vi "scanDeviceStepLogic.vi"(4 "actScan":i32, 6 "actStep":i32) -> (2 "timedOut":bool)   [LabVIEW 2014]
uses:
  Controls/infoHandle.ctl
  Sequencer/trackGlobVar.vi
  scanDeviceGlobalVars.vi
  <vilib>/rvi/Emulation/niFpgaGetClockAttributes.vi
  <vilib>/rvi/Emulation/niFpgaSctlEmulationGetInTimedLoop.vi
  <vilib>/rvi/Emulation/niFpgaEmulationReportErrorSimple.vi
  <vilib>/rvi/Emulation/niFpgaCriticalErrorInLSC.vi
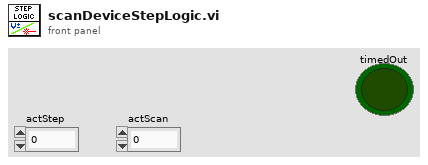
[diagram p1: front panel]
types:
  T1 = typedef "infoHandle.ctl" = enum16{"abortedScan", "stepComplete", "newScan", "newBunch", "preparingStep"}
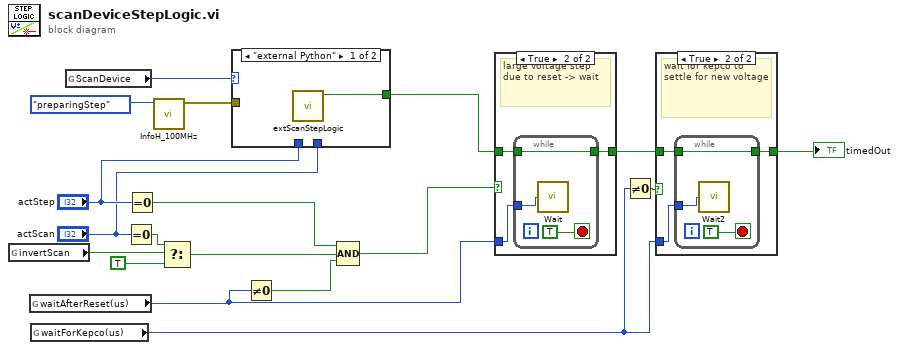
[diagram p0: block diagram]
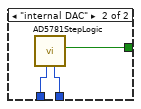
[diagram p2: hidden frame]
diagram:
  n1 = global read "trackGlobVar.vi" "invertScan"() -> (w6:bool)
  n2 = global read "trackGlobVar.vi" "waitAfterReset(us)"() -> (w15:u32)
  n3 = global read "trackGlobVar.vi" "waitForKepco(us)"() -> (w14:u32)
  n4 = global read "scanDeviceGlobalVars.vi" "ScanDevice"() -> (w12:enum16{"internal DAC", "external Python"})
  n5 = Equal To 0?(x="actScan") -> (x = 0?=w9:bool)
  n6 = Equal To 0?(x="actStep") -> (x = 0?=w5:bool)
  n7 = call "InfoH_100MHz.vi"("info"=infoHandle."preparingStep") -> ("Error"=w10:errorcluster)  [unwired: 10 in]
  n8 = Select(t=w9, s=w6, f=TRUE) -> (s? t:f=w7:bool)
  n9 = case shown="\"external Python\"" w12 {
    tunnel: [w19 w22] -> w13
    tunnel: w10 -> [_ _]
    tunnel: "actStep" -> [_ w21]
    tunnel: "actScan" -> [_ w20]
    frame "external Python" {
      n10 = call "extScanStepLogic.vi"() -> ("timedOut"=w19:bool)  [unwired: 11 in]
    }
    frame "internal DAC" {
      n11 = call "AD5781StepLogic.vi"("actScan"=w20, "actStep"=w21) -> ("timedOut"=w22:bool)  [unwired: 9 in]
    }
  }
  n12 = Not Equal To 0?(x=w15) -> (x != 0?=w4:bool)
  n13 = Compound Arithmetic op=AND(w5, w7, w4) -> (w3:bool)
  n14 = case shown="True" w3 {
    tunnel: w13 -> [w23 w26]
    tunnel: [w23 w25] -> w18
    tunnel: w15 -> [_ w24]
    frame False {
    }
    frame True {
      # "large voltage step due to reset -> wait"
      n15 = while {
        tunnel: w26 -> [w28]
        tunnel: [w28] -> w25
        tunnel: w24 -> [w27]
        stop <- TRUE stop-if-true
        n16 = call "Wait"("Count(uSec)"=w27) -> ()  [unwired: 1 out]
      }
    }
  }
  n17 = Not Equal To 0?(x=w14) -> (x != 0?=w17:bool)
  n18 = case shown="True" w17 {
    tunnel: w18 -> [w30 w33]
    tunnel: [w30 w32] -> w16
    tunnel: w14 -> [_ w31]
    frame False {
    }
    frame True {
      # "wait for kepco to settle for new voltage"
      n19 = while {
        tunnel: w33 -> [w35]
        tunnel: [w35] -> w32
        tunnel: w31 -> [w34]
        stop <- TRUE stop-if-true
        n20 = call "Wait2"("Count(uSec)"=w34) -> ()  [unwired: 1 out]
      }
    }
  }
  "timedOut" <- w16
